vi "Timekeeper.vi"   [LabVIEW 2015, in "FPGA Timekeeper.lvlib"]
doc: "The FPGA Timekeeper allows you to synchronize time on your FPGA targets. Place this VI in the top-level VI outside of all block diagram structures."
uses:
  FPGA Timekeeper.lvlib
  <vilib>/rvi/Emulation/niFpgaSctlEmulationGetInTimedLoop.vi
  private/timekeeper locked (g).vi
  <vilib>/rvi/Emulation/niFpgaProcessEmulError.vi
  private/offset from timeref (g).vi
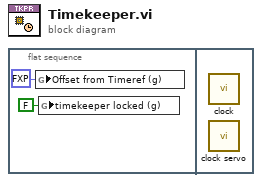
[diagram p0: block diagram]
diagram:
  n1 = flat-sequence {
    frame #0 {
      n2 = global write "offset from timeref (g).vi" "Offset from Timeref (g)"(fxp<+/-,18,18> 0.0 ("Offset from Timeref (g)")) -> ()
      n3 = global write "timekeeper locked (g).vi" "timekeeper locked (g)"(FALSE ("timekeeper locked (g)")) -> ()
    }
    frame #1 {
      n4 = call "clock.vi"() -> ()  [unwired: 12 in]
      n5 = call "clock servo.vi"() -> ()  [unwired: 12 in]
    }
  }
